vi "add_entry.vi"(0 "Active Analog Data In":T2[](array[typedef]), 5 "Add-on Data":T1, 11 "error in":errorcluster) -> (4 "Active Analog Data Out":T2[](array[typedef]), 15 "error out":errorcluster)   [LabVIEW 2017]
uses:
  analog_data.ctl
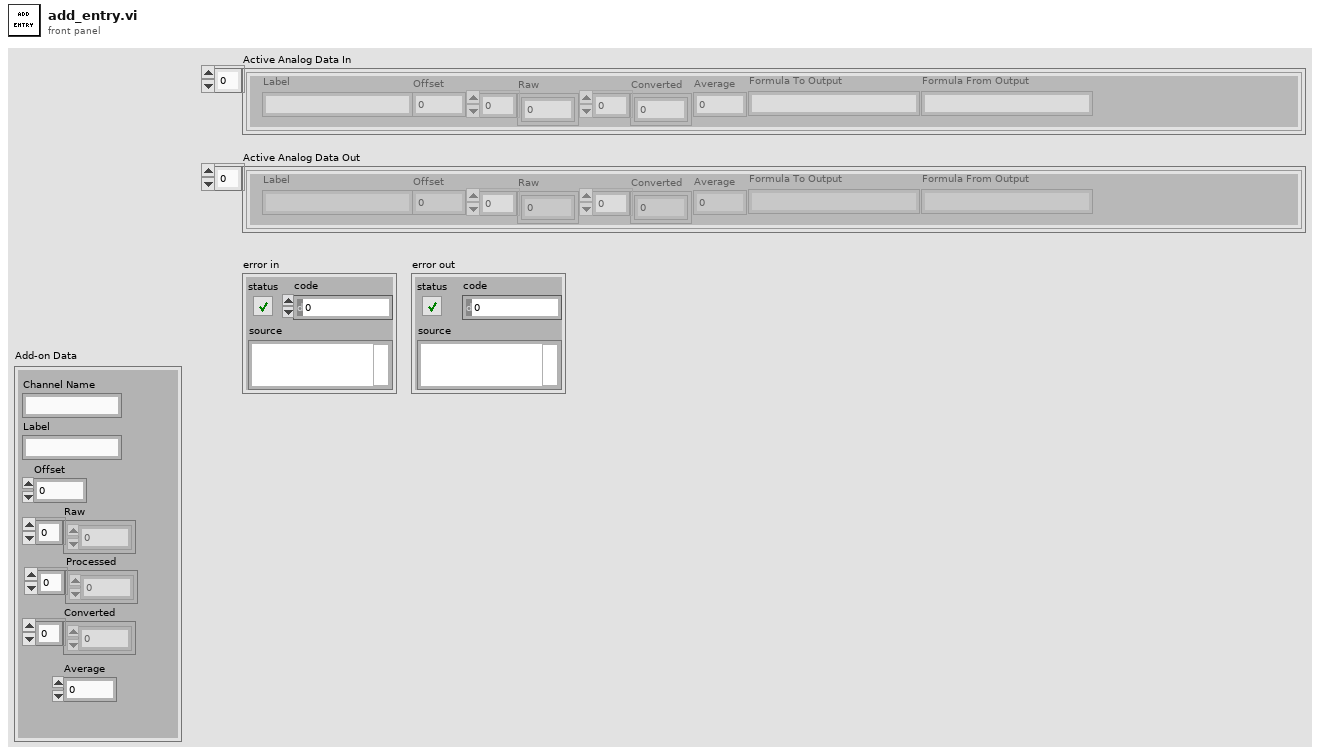
[diagram p1: front panel]
types:
  T1 = cluster{"Channel Name":string, "Label":string, "Offset":dbl, "Raw":dbl[], "Processed":dbl[], "Converted":dbl[], "Average":dbl}
  T2 = typedef "analog_data.ctl" = cluster{"Label":string, "Offset":dbl, "Raw":dbl[], "Converted":dbl[], "Average":dbl, "Formula To Output":string, "Formula From Output":string}
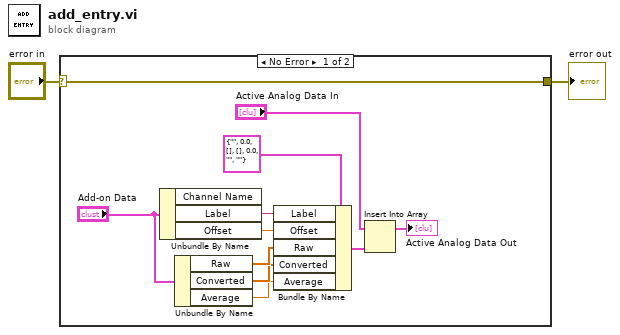
[diagram p0: block diagram]
diagram:
  n1 = case shown="No Error" "error in" {
    selector: "error in" -> [w3 w14]
    tunnel: [w3 w14] -> w1
    frame No Error {
      n2 = Unbundle By Name("Add-on Data") -> ("Label"=w10:string, "Offset"=w9:dbl)  [unwired: 1 out]
      n3 = Unbundle By Name("Add-on Data") -> ("Raw"=w7:dbl[], "Converted"=w6:dbl[], "Average"=w5:dbl)
      n4 = Bundle By Name(cluster=T2 {"Label"="", "Offset"=0.0, "Raw"=[], "Converted"=[], "Average"=0.0, "Formula To Output"="", "Formula From Output"=""} ("Analog Data"), "Label"=w10, "Offset"=w9, "Raw"=w7, "Converted"=w6, "Average"=w5) -> (w4:T2)
      n5 = Insert Into Array(array="Active Analog Data In", new element=w4) -> (→"Active Analog Data Out":T2[])  [unwired: 1 in]
    }
    frame Error {
    }
  }
  "error out" <- w1
